vi "PCM Attribute Set YScale.vi"(8 "error in (no error)":errorcluster caption="错误输入（无错误）", 10 "Y标尺.范围":T1 caption="范围", 11 "PCM PanelSplit 输入":refnum<class "PCM PanelSplit.lvclass"> caption="DNL_LabVIEW Object in") -> (0 "error out":errorcluster caption="错误输出", 3 "PCM PanelSplit 输出":refnum<class "PCM PanelSplit.lvclass"> caption="DNL_LabVIEW Object out")   [LabVIEW 2016, in "PCM PanelSplit.lvclass"]
uses:
  PCM PanelSplit.lvclass
  <vilib>/Utility/miscctls.llb/LVRangeTypeDef.ctl
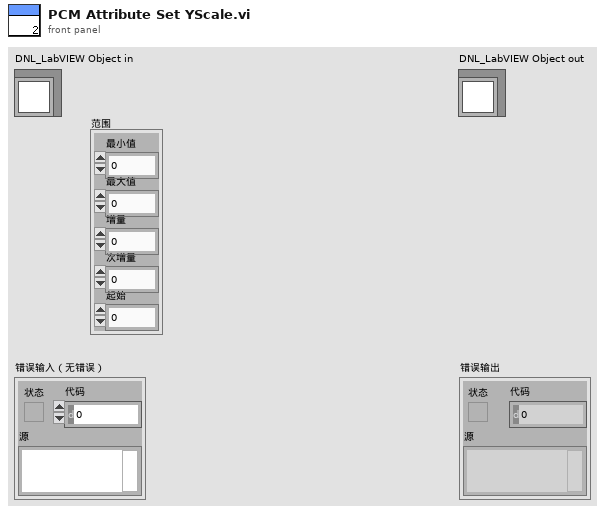
[diagram p1: front panel]
types:
  T1 = typedef "LVRangeTypeDef.ctl" = cluster{"Minimum":dbl, "Maximum":dbl, "Increment":dbl, "Minor Increment":dbl, "Start":dbl}
  T2 = typedef "PCM PanelSplit.lvclass/Display Config.ctl" = cluster{"Display Mode":T3, "ChTag[]":string[], "window":T4, "Range":T1}
  T3 = typedef "PCM PanelSplit.lvclass/Display Mode.ctl" = enum16{"时域", "频谱", "功率谱"}
  T4 = typedef "NI_AALPro.lvlib/windowTd.ctl" = u32
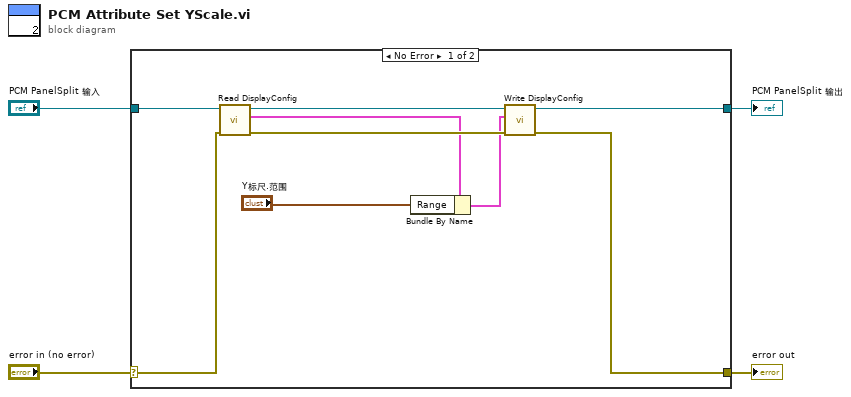
[diagram p0: block diagram]
diagram:
  n1 = case shown="No Error" "error in (no error)" {
    selector: "error in (no error)" -> [w10 w15]
    tunnel: [w8 w15] -> w3
    tunnel: [w11 w14] -> w1
    tunnel: "PCM PanelSplit 输入" -> [w13 w14]
    frame No Error {
      n2 = call "Read DisplayConfig.vi"("error in"=w10, "PCM PanelSplit 输入"=w13) -> ("error out"=w9:errorcluster, "Display Config"=w7:T2, "PCM PanelSplit 输出"=w12:refnum<class "PCM PanelSplit.lvclass">)  [unwired: 7 in]
      n3 = Bundle By Name(cluster=w7, "Range"="Y标尺.范围") -> (w6:T2)
      n4 = call "Write DisplayConfig.vi"("error in"=w9, "Display Config"=w6, "PCM PanelSplit 输入"=w12) -> ("error out"=w8:errorcluster, "PCM PanelSplit 输出"=w11:refnum<class "PCM PanelSplit.lvclass">)  [unwired: 7 in]
    }
    frame Error {
    }
  }
  "error out" <- w3
  "PCM PanelSplit 输出" <- w1
